vi "LogData_Command.vi"(7 "Motores_Queue":T1, 8 "error_in":errorcluster, 9 "array":u8[](array[numeric]), 10 "DataLogger_queue_in":refnum<queue>, 11 "has program started?":bool=TRUE) -> (0 "error out":errorcluster, 2 "DataLogger_Queue_out":refnum<queue>)   [LabVIEW 2026]
uses:
  Control/Ctrl_DataLoggerQueue.ctl
  Ctrl_Estados.ctl
  Control/Ctr_Enc_Values.ctl
  Control/Ctrl_Motores_Valores.ctl
  Control/Ctrl_Errores.ctl
  Control/Ctrl_EscrituraComandos.ctl
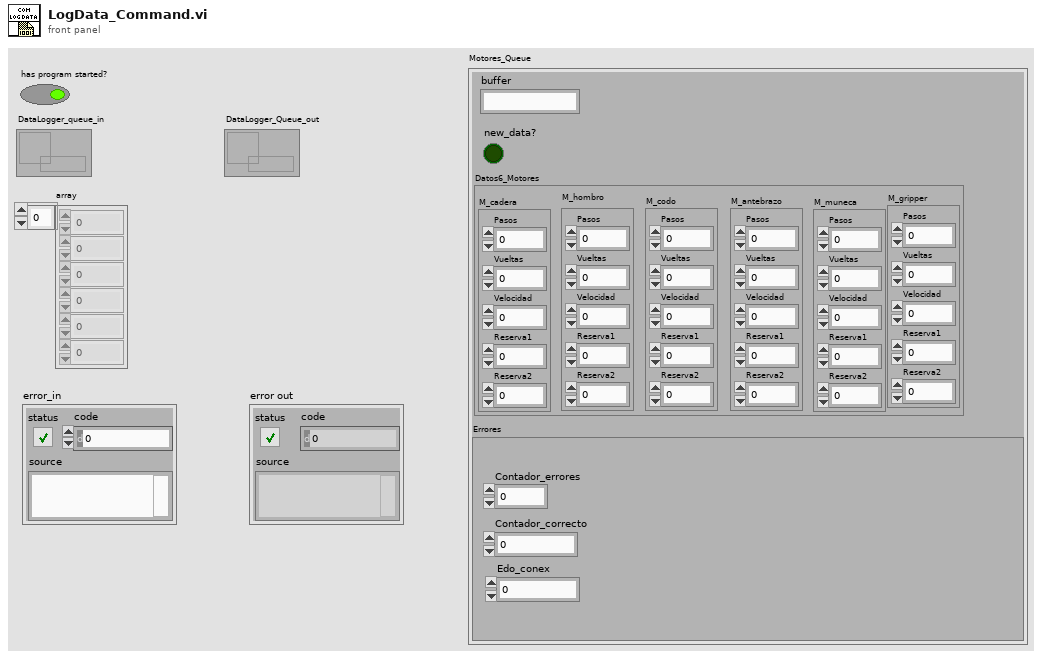
[diagram p1: front panel]
types:
  T1 = typedef "Ctr_Enc_Values.ctl" = cluster{"buffer":string, "Datos6_Motores":cluster{"M_cadera":T2, "M_hombro":T2, "M_codo":T2, "M_antebrazo":T2, "M_muneca":T2, "M_gripper":T2}, "Errores":T3, "new_data?":bool}
  T2 = typedef "Ctrl_Motores_Valores.ctl" = cluster{"Pasos":i32, "Vueltas":i16, "Velocidad":i16, "Reserva1":u8, "Reserva2":u8}
  T3 = typedef "Ctrl_Errores.ctl" = cluster{"Contador_correcto":u32, "Contador_errores":u32, "Edo_conex":u32}
  T4 = typedef "Ctrl_DataLoggerQueue.ctl" = cluster{"IncioPrograma":bool, "Estado":T5, "Enc_values":T1, "Com_Escribir":T6}
  T5 = typedef "Ctrl_Estados.ctl" = enum16{"LogData", "Idle", "Stop", "Log_Data_All", "Start", "Write", "Reconnect"}
  T6 = typedef "Ctrl_EscrituraComandos.ctl" = enum16{"MOVE_10", "HOME_TO"}
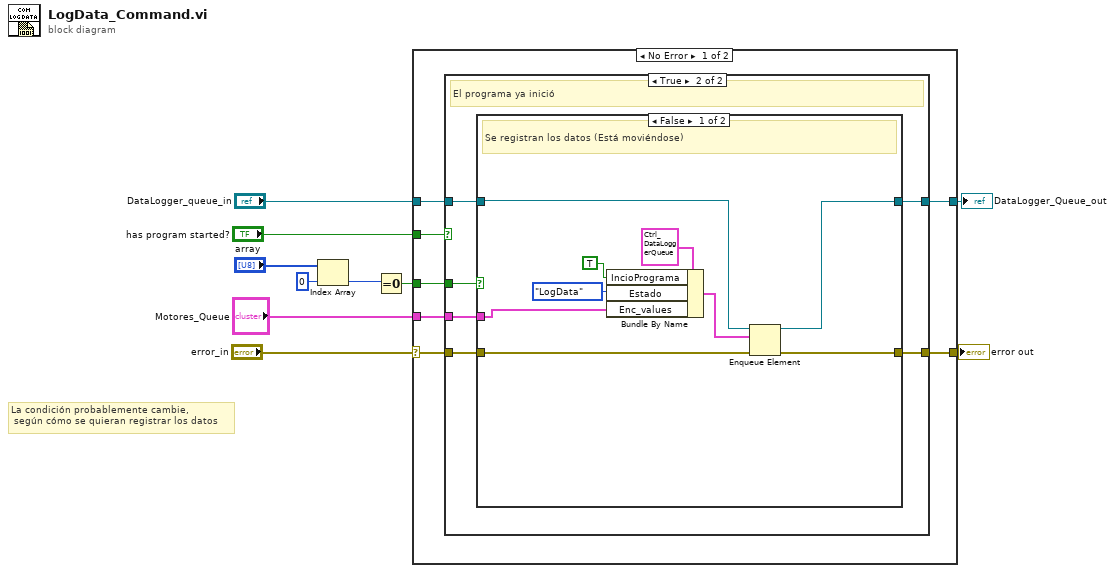
[diagram p0: block diagram]
diagram:
  # "La condición probablemente cambie,\n según cómo se quieran registrar los datos"
  n1 = Index Array(array="array", index=0) -> (element=w8:u8)
  n2 = Equal To 0?(x=w8) -> (x = 0?=w9:bool)
  n3 = case shown="No Error" "error_in" {
    selector: "error_in" -> [w14 w37]
    tunnel: w9 -> [w17 _]
    tunnel: "DataLogger_queue_in" -> [w16 w38]
    tunnel: [w15 w38] -> w5
    tunnel: [w13 w37] -> w3
    tunnel: "has program started?" -> [w12 _]
    tunnel: "Motores_Queue" -> [w11 _]
    frame No Error {
      n4 = case shown="True" w12 {
        tunnel: w17 -> [_ w25]
        tunnel: w16 -> [w19 w24]
        tunnel: [w19 w23] -> w15
        tunnel: w14 -> [w18 w22]
        tunnel: [w18 w21] -> w13
        tunnel: w11 -> [_ w20]
        frame False {
          # "El programa no ha iniciado"
        }
        frame True {
          # "El programa ya inició"
          n5 = case shown="False" w25 {
            tunnel: [w30 w35] -> w21
            tunnel: w24 -> [w29 w36]
            tunnel: [w28 w36] -> w23
            tunnel: w22 -> [w27 w35]
            tunnel: w20 -> [w26 _]
            frame False {
              # "Se registran los datos (Está moviéndose)"
              n6 = Bundle By Name(cluster=T4 {"IncioPrograma"=FALSE, "Estado"=enum."Start", "Enc_values"={"buffer"="", "Datos6_Motores"={"M_cadera"={"Pasos"=0, "Vueltas"=0, "Velocidad"=0, "Reserva1"=0, "Reserva2"=0}, "M_hombro"={"Pasos"=0, "Vueltas"=0, "Velocidad"=0, "Reserva1"=0, "Reserva2"=0}, "M_codo"={"Pasos"=0, "Vueltas"=0, "Velocidad"=0, "Reserva1"=0, "Reserva2"=0}, "M_antebrazo"={"Pasos"=0, "Vueltas"=0, "Velocidad"=0, "Reserva1"=0, "Reserva2"=0}, "M_muneca"={"Pasos"=0, "Vueltas"=0, "Velocidad"=0, "Reserva1"=0, "Reserva2"=0}, "M_gripper"={"Pasos"=0, "Vueltas"=0, "Velocidad"=0, "Reserva1"=0, "Reserva2"=0}}, "Errores"={"Contador_correcto"=0, "Contador_errores"=0, "Edo_conex"=0}, "new_data?"=FALSE}, "Com_Escribir"=enum."MOVE_10"} ("datalogger_cluster"), "IncioPrograma"=TRUE, "Estado"=Ctrl_Estados."LogData", "Enc_values"=w26) -> (w31:T4)
              n7 = Enqueue Element(queue=w29, element=w31, error in (no error)=w27) -> (queue out=w28:refnum<queue>, error out=w30:errorcluster)  [unwired: 1 in, 1 out]
            }
            frame True {
              # "Estado == 0"
            }
          }
        }
      }
    }
    frame Error {
    }
  }
  "DataLogger_Queue_out" <- w5
  "error out" <- w3
